vi "Run.vi"(8 "error in (no error)":errorcluster, 9 "s on last turn":dbl, 10 "Maze (0: Empty, -1: Enemy. >0: Teammate":i32[][](array[numeric]), 11 "Scout In":refnum<class "Coward.lvclass">) -> (0 "error out":errorcluster, 1 "Direction":T1, 2 "Action":T2, 3 "Scout Out":refnum<class "Coward.lvclass">, 4 "Replicated":refnum<class "Square.lvclass">)   [LabVIEW 2015, in "Coward.lvclass"]
uses:
  Coward.lvclass
  Formics/Formics.lvclass
  Formics/Attack Options.ctl
  Type Defs/Action Enum.ctl
  Square/Square.lvclass
  Type Defs/Direction Enum.ctl
panel:
  in  "Status":string
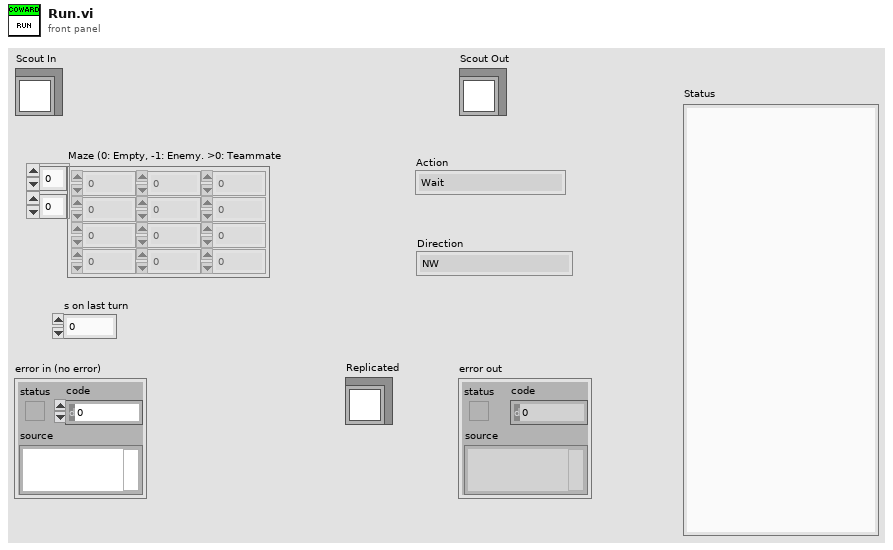
[diagram p1: front panel]
types:
  T1 = typedef "Square.lvclass/Direction Enum.ctl" = enum16{"NW", "N", "NE", "E", "SE", "S", "SW", "W"}
  T2 = typedef "Square.lvclass/Action Enum.ctl" = enum16{"Wait", "Move", "Attack", "Replicate"}
  T3 = typedef "Formics.lvclass/Attack Options.ctl" = enum16{"Attack", "Run", "Distract"}
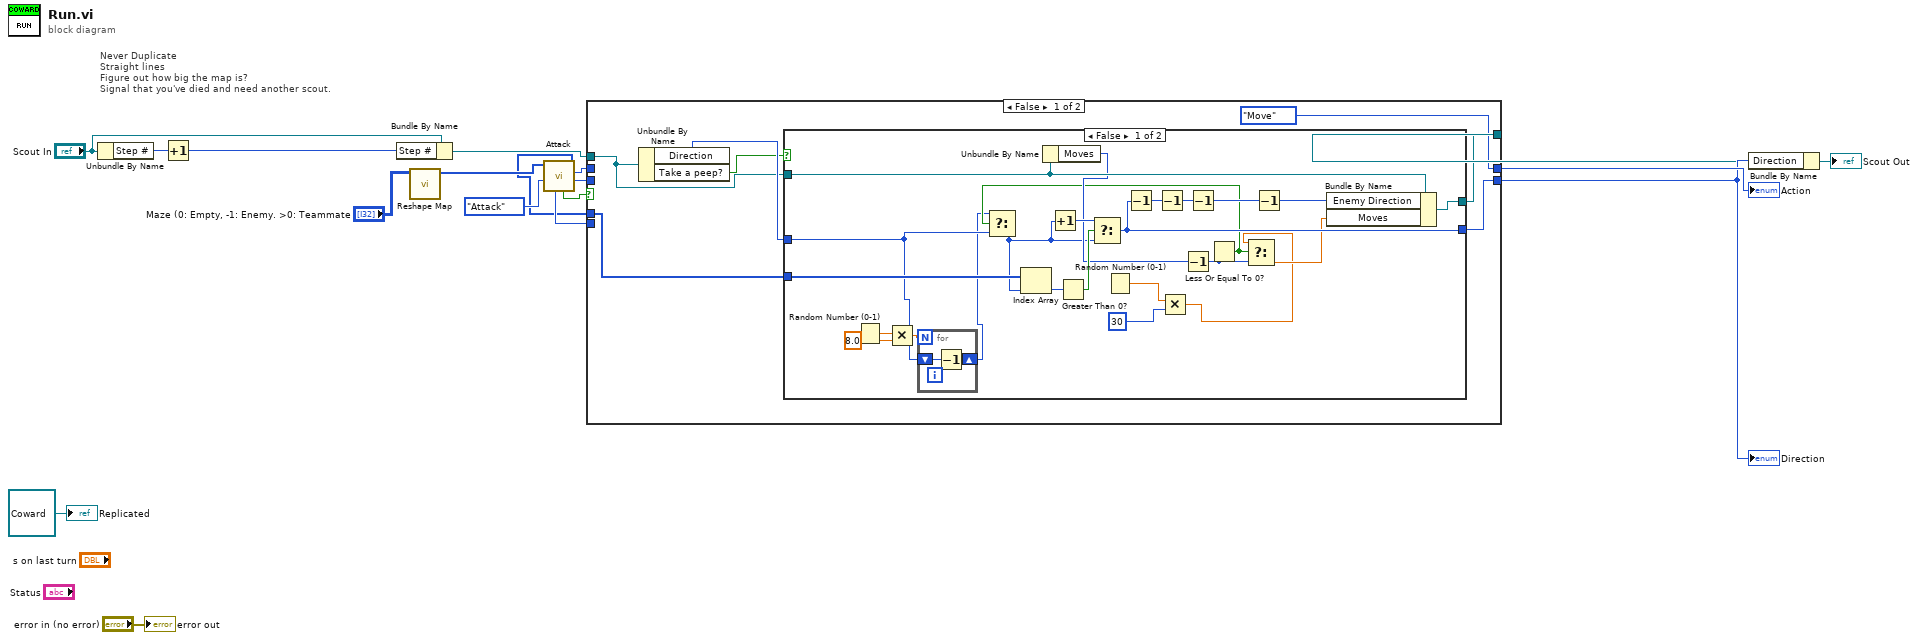
[diagram p0: block diagram]
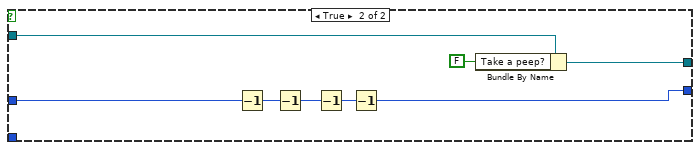
[diagram p2: hidden frame]
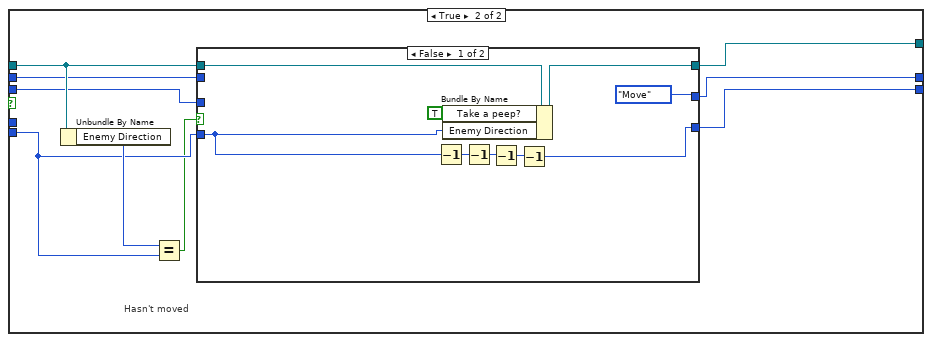
[diagram p3: hidden frame]
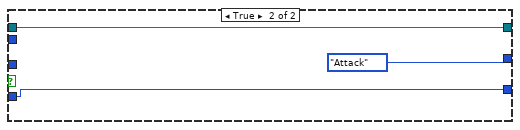
[diagram p4: hidden frame]
diagram:
  # "Never Duplicate\nStraight lines\nFigure out how big the map is?\nSignal that you've died and need another scout."
  n1 = Unbundle By Name("Scout In") -> ("Step #"=w6:i32)
  n2 = Increment(x=w6) -> (x+1=w15:i32)
  n3 = Bundle By Name(cluster="Scout In", "Step #"=w15) -> (w3:refnum<class "Coward.lvclass">)
  n4 = call "Reshape Map.vi"("Maze (0: Empty, -1: Enemy. >0: Teammate"="Maze (0: Empty, -1: Enemy. >0: Teammate") -> ("Map"=w2:i32[])  [unwired: 9 in, 1 out]
  n5 = call "Attack.vi"("Attack?"=Attack_Options."Attack", "Maze (0: Empty, -1: Enemy. >0: Teammate"=w2) -> ("Direction"=w8:i32, "Action"=w10:T2, "Maze (0: Empty, -1: Enemy. >0: Teammate 2"=w1:i32[], "Enemy Found?"=w11:bool, "Enemy Direction"=w4:i32)  [unwired: 4 in, 1 out]
  n6 = case shown="False" w11 {
    tunnel: w10 -> [_ w65]
    tunnel: [Action_Enum."Move" ("Action") w64] -> w9
    tunnel: w8 -> [_ w66]
    tunnel: [w24 w63] -> w7
    tunnel: w1 -> [w23 _]
    tunnel: w3 -> [w20 w67]
    tunnel: [w19 w68] -> w5
    tunnel: w4 -> [_ w61]
    frame False {
      n7 = Unbundle By Name(w20) -> ("Direction"=w22:T1, "Take a peep?"=w21:bool)
      n8 = case shown="False" w21 {
        tunnel: [w44 w55] -> w24
        tunnel: w23 -> [w49 _]
        tunnel: w22 -> [w30 w59]
        tunnel: w20 -> [w39 w54]
        tunnel: [w45 w53] -> w19
        frame False {
          n9 = Random Number (0-1)() -> (number: 0 to 1=w35:dbl)
          n10 = Multiply(x=w35, y=8.0) -> (x*y=w31:dbl)
          n11 = for {
            N: w31 -> [_]
            shift-right: [w50] -> w29
            shift-left: w30 -> [w51]
            n12 = Decrement(x=w51) -> (x-1=w50:T1)
          }
          n13 = Unbundle By Name(w39) -> ("Moves"=w38:i32)
          n14 = Random Number (0-1)() -> (number: 0 to 1=w28:dbl)
          n15 = Multiply(x=w28, y=30 ("t")) -> (x*y=w26:dbl)
          n16 = Decrement(x=w38) -> (x-1=w36:i32)
          n17 = Less Or Equal To 0?(x=w36) -> (x <= 0?=w32:bool)
          n18 = Select(t=w29, s=w32, f=w30) -> (s? t:f=w33:T1)
          n19 = Index Array(array=w49, index=w33) -> (element=w48:i32)
          n20 = Increment(x=w33) -> (x+1=w46:T1)
          n21 = Greater Than 0?(x=w48) -> (x > 0?=w47:bool)
          n22 = Select(t=w46, s=w47, f=w33) -> (s? t:f=w44:T1)
          n23 = Decrement(x=w44) -> (x-1=w43:T1)
          n24 = Decrement(x=w43) -> (x-1=w42:T1)
          n25 = Decrement(x=w42) -> (x-1=w41:T1)
          n26 = Select(t=w26, s=w32, f=w36) -> (s? t:f=w37:dbl)
          n27 = Decrement(x=w41) -> (x-1=w40:T1)
          n28 = Bundle By Name(cluster=w39, "Enemy Direction"=w40, "Moves"=w37) -> (w45:refnum<class "Coward.lvclass">)
        }
        frame True {
          n29 = Decrement(x=w59) -> (x-1=w58:T1)
          n30 = Decrement(x=w58) -> (x-1=w57:T1)
          n31 = Decrement(x=w57) -> (x-1=w56:T1)
          n32 = Decrement(x=w56) -> (x-1=w55:T1)
          n33 = Bundle By Name(cluster=w54, "Take a peep?"=FALSE) -> (w53:refnum<class "Coward.lvclass">)
        }
      }
    }
    frame True {
      # "Hasn't moved"
      n34 = Unbundle By Name(w67) -> ("Enemy Direction"=w62:T1)
      n35 = Equal?(x=w62, y=w61) -> (x = y?=w60:bool)
      n36 = case shown="False" w60 {
        tunnel: [w77 w80] -> w68
        tunnel: w67 -> [w75 w80]
        tunnel: w66 -> [_ _]
        tunnel: w65 -> [_ _]
        tunnel: [Action_Enum."Move" ("Action") Action_Enum."Attack" ("Action")] -> w64
        tunnel: [w70 w78] -> w63
        tunnel: w61 -> [w71 w78]
        frame False {
          n37 = Decrement(x=w71) -> (x-1=w74:i32)
          n38 = Bundle By Name(cluster=w75, "Take a peep?"=TRUE, "Enemy Direction"=w71) -> (w77:refnum<class "Coward.lvclass">)
          n39 = Decrement(x=w74) -> (x-1=w72:i32)
          n40 = Decrement(x=w72) -> (x-1=w73:i32)
          n41 = Decrement(x=w73) -> (x-1=w70:i32)
        }
        frame True {
        }
      }
    }
  }
  "Action" <- w9
  "Direction" <- w7
  n42 = Bundle By Name(cluster=w5, "Direction"=w7) -> (→"Scout Out":refnum<class "Coward.lvclass">)
  "error out" <- "error in (no error)"
  "Replicated" <- refnum<class "Coward.lvclass"> refnum ("Replicated")
